vi "Get Pin Status.vi"(8 "error in (no error)":errorcluster, 9 "Pin":dbl, 10 "Port":dbl, 11 "Serial device in":refnum<class "Serial device.lvclass">) -> (0 "error out":errorcluster, 3 "Serial device out":refnum<class "Serial device.lvclass">)   [LabVIEW 2020, in "Serial device.lvclass"]
doc: "Metodo del papá dynamic dispatch para mandar la cadena del estado de un pin del dispositivo serial."
uses:
  Serial device.lvclass
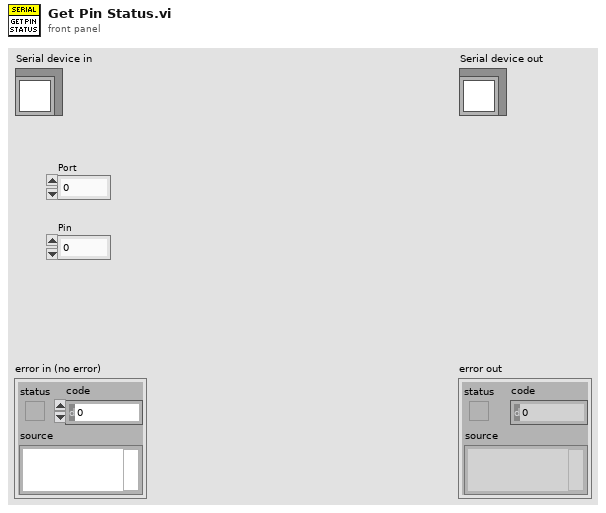
[diagram p1: front panel]
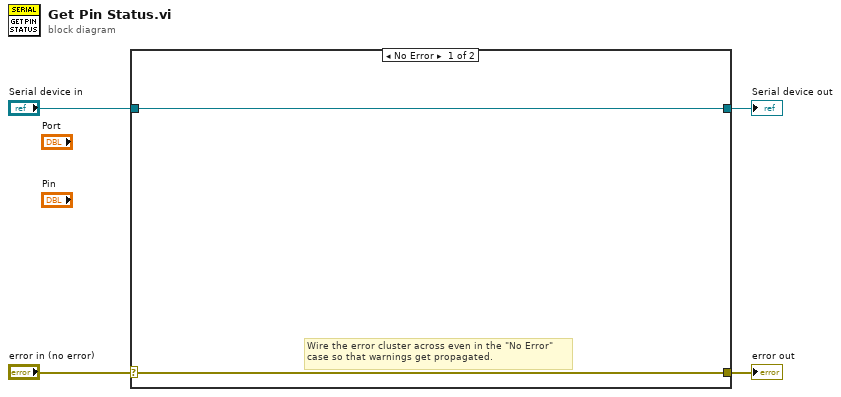
[diagram p0: block diagram]
diagram:
  n1 = case shown="No Error" "error in (no error)" {
    selector: "error in (no error)" -> [w5 w8]
    tunnel: [w5 w8] -> w3
    tunnel: [w6 w7] -> w1
    tunnel: "Serial device in" -> [w6 w7]
    frame No Error {
      # "Wire the error cluster across even in the \"No Error\"\ncase so that warnings get propagated."
    }
    frame Error {
    }
  }
  "error out" <- w3
  "Serial device out" <- w1
